vi "Open Preferences File.vi"(11 "Operation":enum16{"Load", "Save"}(ring)=2) -> (0 "error out":errorcluster, 3 "File refnum out":T1)   [LabVIEW 2013]
uses:
  <vilib>/Utility/config.llb/Config Data RefNum.ctl
  <vilib>/Utility/config.llb/NI_LVConfig.lvlib
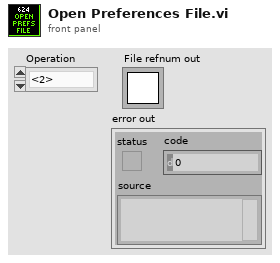
[diagram p1: front panel]
types:
  T1 = typedef "NI_LVConfig.lvlib/Config Data RefNum.ctl" = refnum<k1>
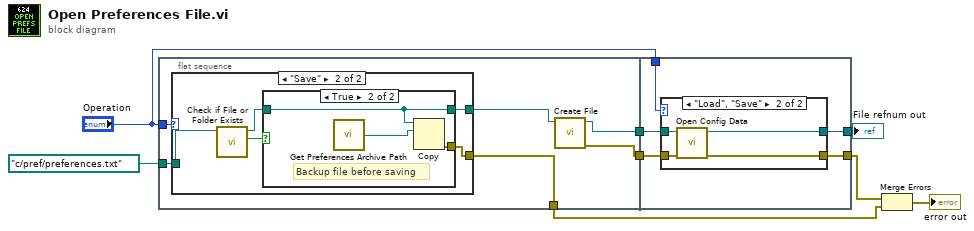
[diagram p0: block diagram]
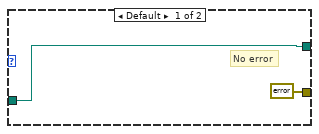
[diagram p2: hidden frame]
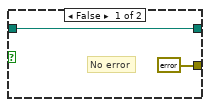
[diagram p3: hidden frame]
diagram:
  n1 = flat-sequence {
    tunnel: "Operation" -> [w14]
    tunnel: path "c:/pref/preferences.txt" ("configuration file path") -> [w13]
    tunnel: [w10] -> w5
    tunnel: [w11] -> w4
    tunnel: [w9] -> w1
    tunnel: [w31] -> w8
    tunnel: "Operation" -> [w30]
    tunnel: w5 -> [w29]
    tunnel: [w28] -> w2
    tunnel: w4 -> [w27]
    frame #0 {
      n2 = case shown="\"Save\"" w14 {
        tunnel: w13 -> [w15 w19]
        tunnel: [errorcluster {"status"=FALSE, "code"=0, "source"=""} ("error out") w21] -> w9
        tunnel: [w15 w17] -> w12
        frame Default {
          # "No error"
        }
        frame "Save" {
          n3 = call <vilib>:"Check if File or Folder Exists.vi"("path"=w19) -> ("file or folder exists?"=w20:bool, "dup path"=w18:path)  [unwired: 8 in, 1 out]
          n4 = case shown="True" w20 {
            tunnel: [errorcluster {"status"=FALSE, "code"=0, "source"=""} ("error out") w26] -> w21
            tunnel: w18 -> [w22 w25]
            tunnel: [w22 w25] -> w17
            frame False {
              # "No error"
            }
            frame True {
              # "Backup file before saving"
              n5 = call "Get Preferences Archive Path.vi"() -> ("path"=w24:path)  [unwired: 1 in]
              n6 = Copy(10:w24, 11:w25) -> (0:w26:errorcluster)  [unwired: 3 in, 2 out]
            }
          }
        }
      }
      n7 = call "Create File.vi"("path"=w12) -> ("error out"=w10:errorcluster, "path out"=w11:path)  [unwired: 9 in]
    }
    frame #1 {
      n8 = case shown="\"Load\", \"Save\"" w30 {
        tunnel: [_ w36] -> w31
        tunnel: w29 -> [w32 w35]
        tunnel: [w32 w34] -> w28
        tunnel: w27 -> [_ w33]
        frame Default {
          # "No Preferences needed\n(use default value)"
        }
        frame "Load", "Save" {
          n9 = call <vilib>:"Open Config Data.vi"("error in (no error)"=w35, "configuration file path"=w33) -> ("error out"=w34:errorcluster, "refnum"=w36:T1)  [unwired: 7 in, 1 out]
        }
      }
    }
  }
  n10 = Merge Errors(w2, w1) -> (→"error out":errorcluster)
  "File refnum out" <- w8
